vi "PicoScope6000ExampleStreaming.vi"() -> ()   [LabVIEW 2010]
doc: "This example demonstrates how to use the PicoScope Labview library to stream data from a PicoScope 5000 Series Device"
uses:
  PicoScope6000Lib/PicoScope6000AnalogChannelSettings.ctl
panel:
  in  "Write to file":bool
  in  "Trigger Settings":T1={"Trigger Enabled"=FALSE, "Trigger Source"=enum."Channel A", "Trigger Threshold (Volts)"=0.0, "Trigger Direction"=2, "Trigger Delay (samples)"=0, "Auto Trigger Time (ms)"=1000} {"Trigger Direction" items=["Rising"=2, "Falling"=3]}
  in  "error in (no error)":errorcluster
  out "Device Info":T2
  in  "Channel A Settings":T3={"Enabled"=TRUE, "Coupling"=1, "Range"=6, "Analogue Offset"=0.0, "Bandwidth"=0} {"Bandwidth" items=["Full", "20 MHz"]; "Range" items=["10 mV", "20 mV", "50 mV", "100 mV", "200 mV", "500 mV", "1 V", "2 V", "5 V", "10 V", "20 V", "50 V ", "100 V"]; "Coupling" items=["AC", "DC 1 MOhm", "DC 50 Ohm"]}
  out "Analog Channels":T4(graph)
  out "Raw Sample Interval (sec)":dbl=1.0000000130088963e-06 format="%#.5p"
  out "Max ADC value":i16=32512
  out "Chunk time":u32
  out "Elapsed time":dbl
  in  "Data file":path=path "PicoScope6000ExampleStreaming ChA Data"
  out "size(s)":i32
  out "Queue depth":i32(graph)
  out "queue depth":i32
  in  "Buffer and Transfer Settings":T5={"startIndex"=0, "Samples"=1000000, "Down Sample Ratio"=1, "Down-Sample Mode"=0} {"Down-Sample Mode" items=["None"=0, "Aggregate"=1, "Decimate"=2, "Average"=4]; "Down Sample Ratio" step=1; "Samples" format="%_6p"}
  out "TriggeredAt (In Buffer)":u32 format="%#.6p"
  out "TriggeredAt (Total samples)":u32 format="%#.6p"
  in  "Acquisition Settings":T6={"Auto Stop"=TRUE, "Desired Sample Interval"=1, "Pre-trigger Samples"=0, "Post-trigger Samples"=1000000, "Down-Sample Ratio"=1, "Down-Sample Mode"=0, "Time Units"=3} {"Time Units" items=["Nanoseconds (ns)"=2, "Microseconds (us)"=3, "Milliseconds (ms)"=4, "Seconds (s)"=5]; "Down-Sample Mode" items=["None"=0, "Aggregate"=1, "Decimate"=2, "Average"=4]; "Post-trigger Samples" format="%#.6p"; "Pre-trigger Samples" format="%#_6p"}
  out "Triggered":bool
  out "DownSample Interval (sec)":dbl=1.0000000130088963e-06 format="%#.5p"
  out "Total Samples":u32 format="%#.6p"
  out "Auto Stopped":bool
  in  "Serial Number":string
  in  "Open Using\nSerial Number":bool
  out "Number of Samples per Capture":u32 format="%#.6p"
  in  "Apply  Settings":bool
  in  "stop":bool
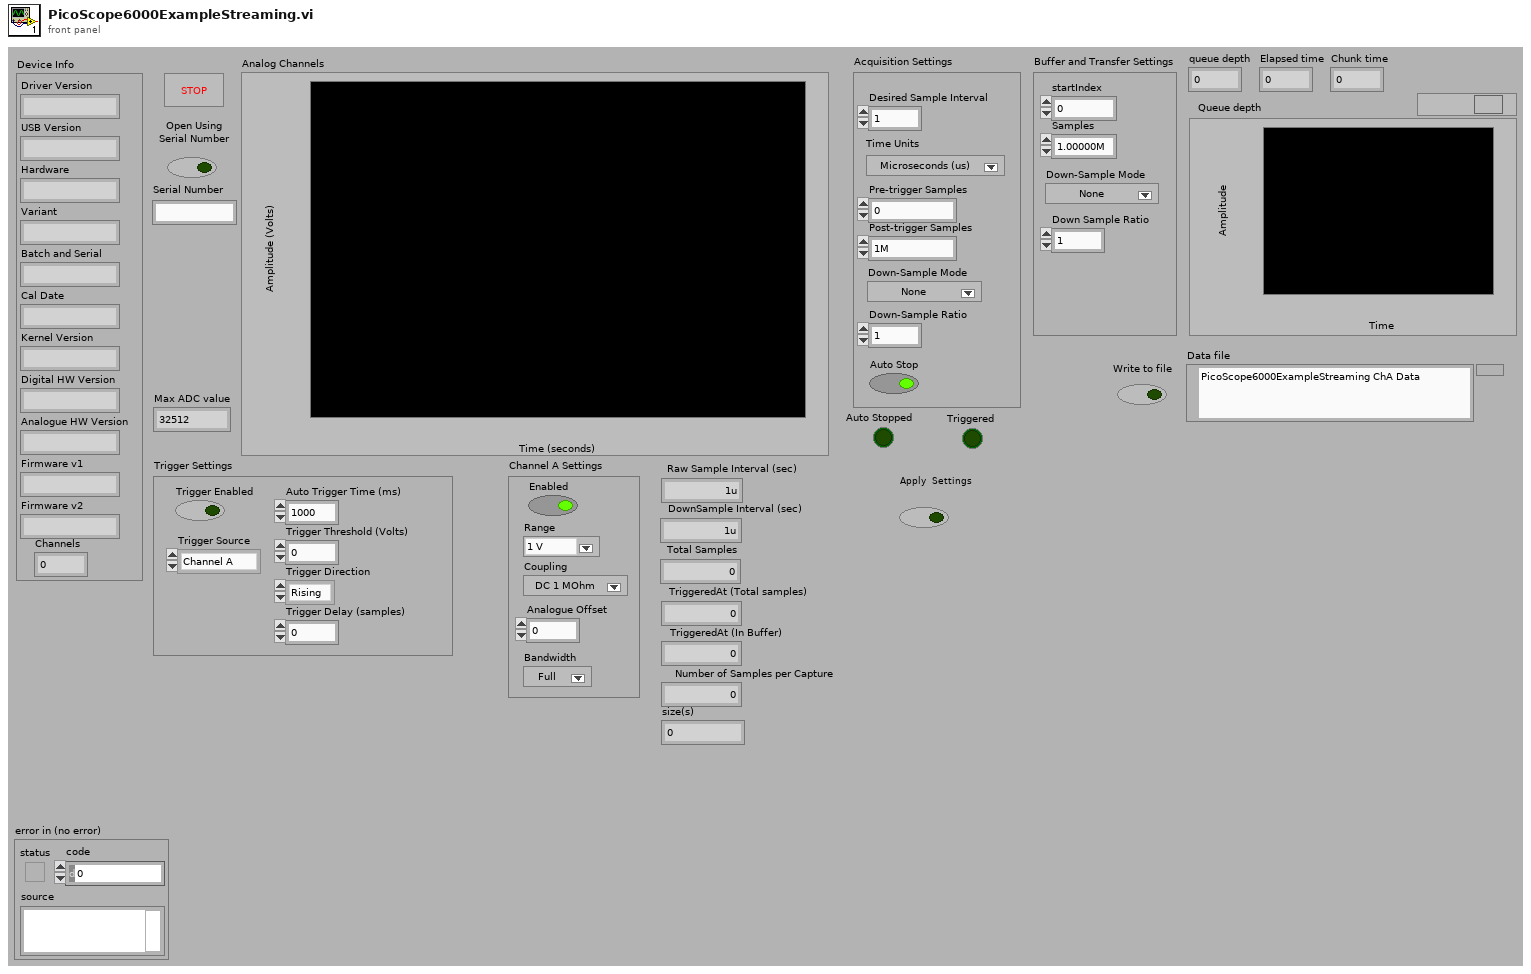
[diagram p1: front panel]
types:
  T1 = cluster{"Trigger Enabled":bool, "Trigger Source":enum32{"Channel A", "Channel B", "Channel C", "Channel D", "External", "Aux."}, "Trigger Threshold (Volts)":dbl, "Trigger Direction":u16, "Trigger Delay (samples)":u32, "Auto Trigger Time (ms)":i16}
  T2 = cluster{"Driver Version":string, "USB Version":string, "Hardware":string, "Variant":string, "Batch and Serial":string, "Cal Date":string, "Kernel Version":string, "Digital HW Version":string, "Analogue HW Version":string, "Firmware v1":string, "Firmware v2":string, "Channels":i16}
  T3 = typedef "PicoScope6000AnalogChannelSettings.ctl" = cluster{"Enabled":bool, "Coupling":u32, "Range":u32, "Analogue Offset":sgl, "Bandwidth":u32}
  T4 = cluster{i32, "DownSample Interval (sec)":dbl, "Data":dbl[]}
  T5 = cluster{"startIndex":u64, "Samples":u64, "Down Sample Ratio":u64, "Down-Sample Mode":u32}
  T6 = cluster{"Auto Stop":bool, "Desired Sample Interval":u32, "Pre-trigger Samples":u32, "Post-trigger Samples":u32, "Down-Sample Ratio":u32, "Down-Sample Mode":i32, "Time Units":u32}
  T7 = enum16{"open", "open or create", "create or replace", "create", "open (read-only)"}
  T8 = cluster{"Enabled":bool, "Coupling":i32, "Range":u16, "Analogue Offset":sgl, "Bandwidth":i32}
  T9 = cluster{"Channel A Buffer":i16[], "Channel B Buffer":i16[], "Channel C Buffer":i16[], "Channel D Buffer":i16[], "Channel E Buffer":i16[], "Channel F Buffer":i16[], "Channel G Buffer":i16[], "Channel H Buffer":i16[], "Port 0":i16[], "Port 1":i16[]}
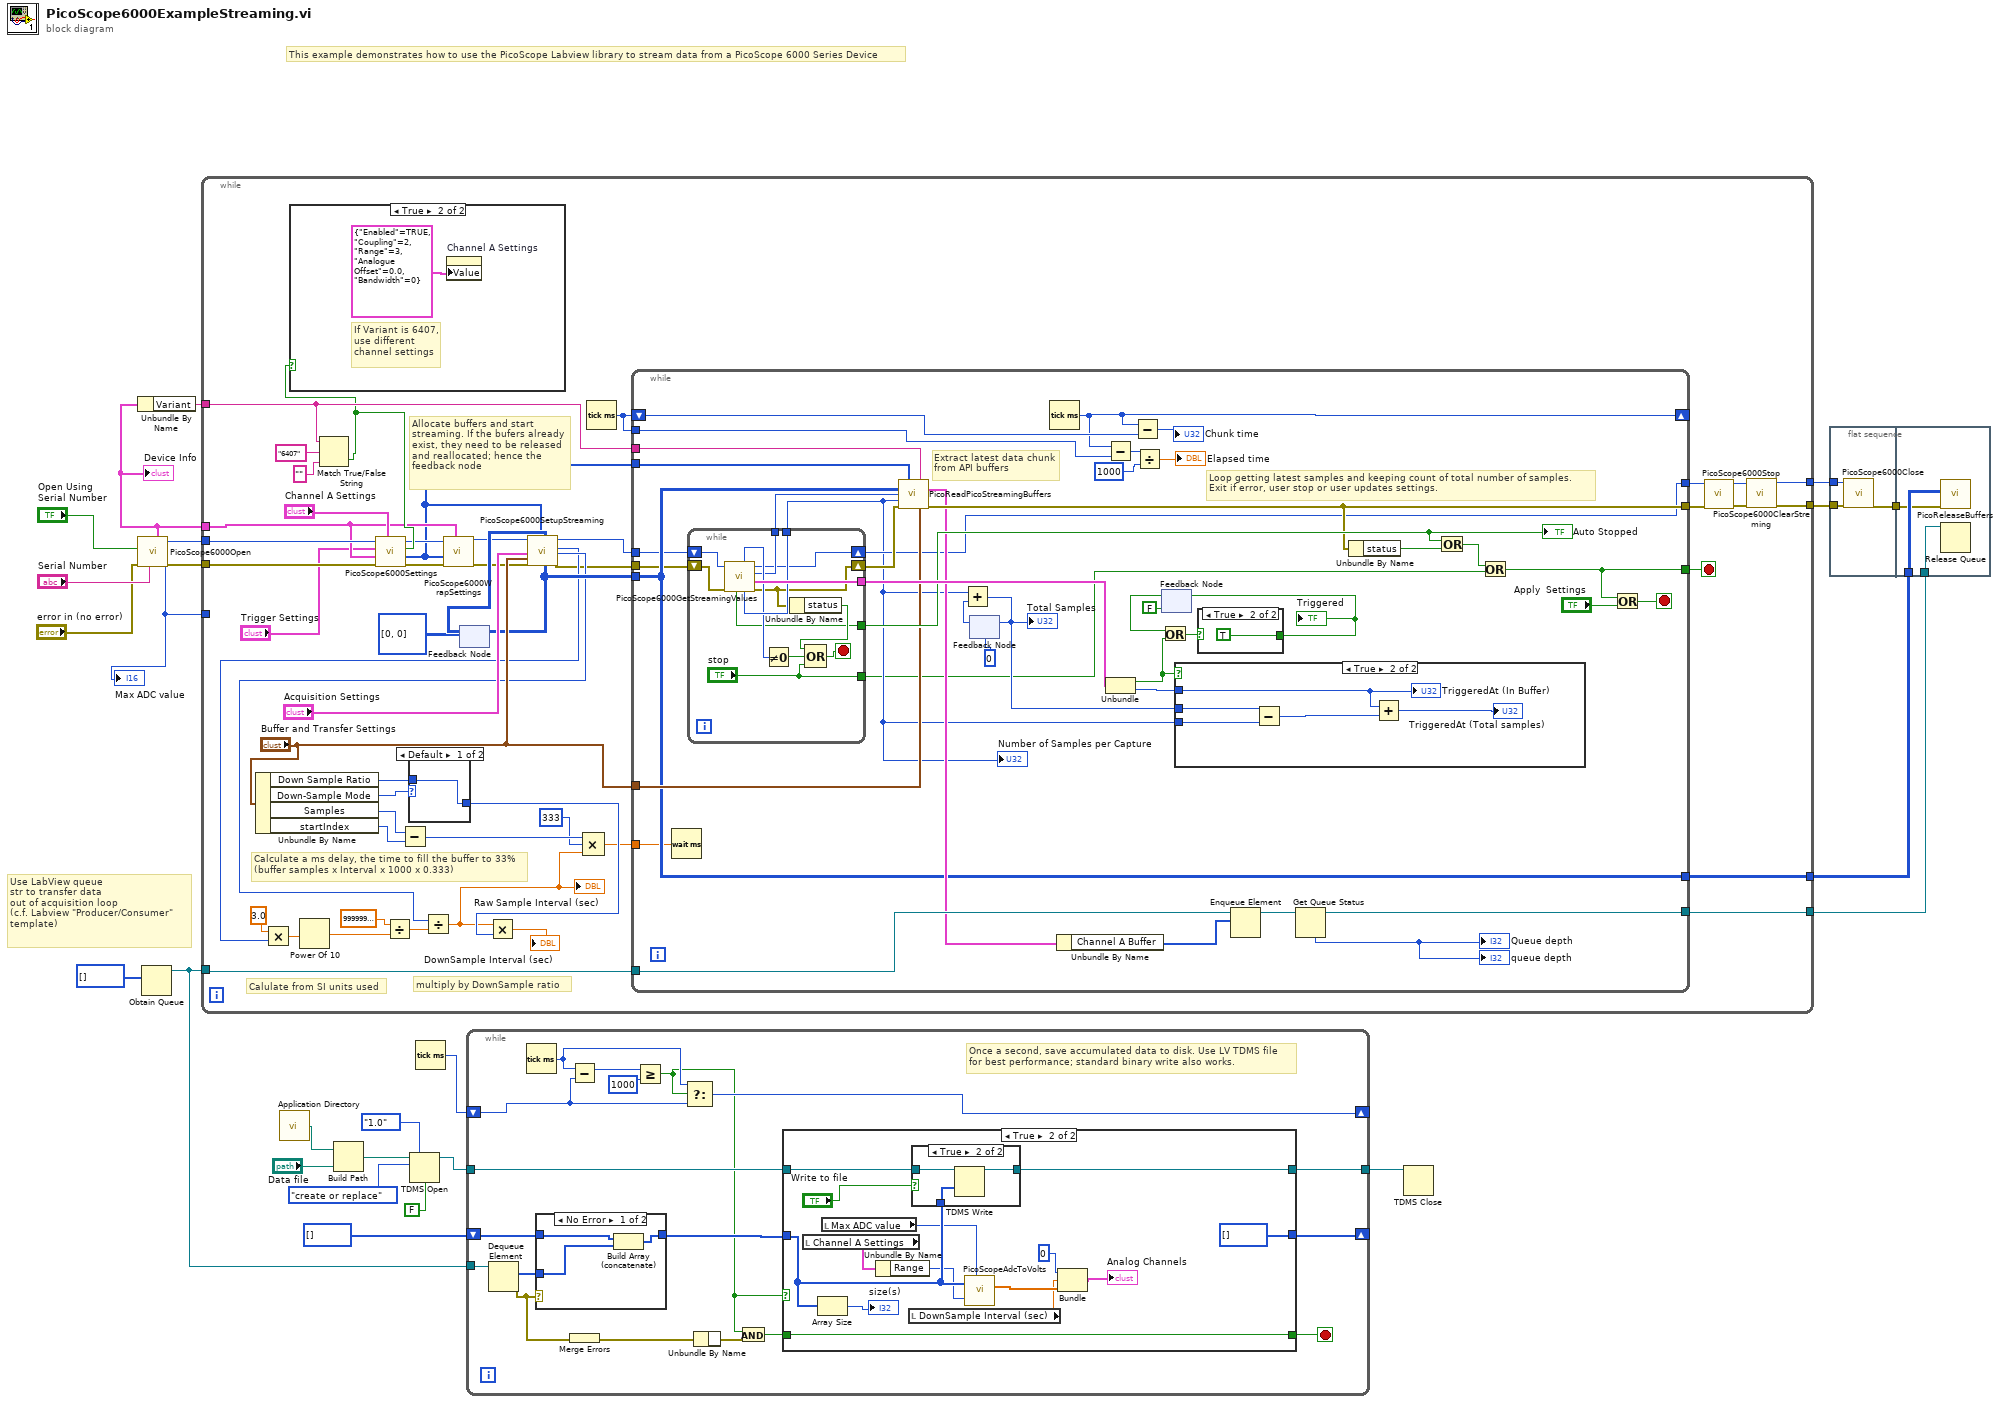
[diagram p0: block diagram]
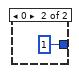
[diagram p6: hidden frame]
diagram:
  # "Use LabView queue\nstr to transfer data\nout of acquisition loop\n(c.f. Labview \"Producer/Consumer\"\ntemplate)"
  # "This example demonstrates how to use the PicoScope Labview library to stream data from a PicoScope 6000 Series Device"
  n1 = call "PicoScope6000Open.vi"("error in (no error)"="error in (no error)", "Serial Number"="Serial Number", "Use Serial Number"="Open Using\nSerial Number") -> ("error out"=w25:errorcluster, "Max Adc value"=w21:i16, "handle"=w24:i16, "Device Info"=w4:T2)  [unwired: 4 in, 1 out]
  "Max ADC value" <- w21
  "Device Info" <- w4
  n2 = Unbundle By Name(w4) -> ("Variant"=w5:string)
  n3 = Obtain Queue(element data type=i16[] [] ("History Data")) -> (queue out=w20:refnum<queue>)  [unwired: 4 in, 2 out]
  n4 = while {
    tunnel: [w27] -> w19
    tunnel: w25 -> [w44]
    tunnel: w24 -> [w43]
    tunnel: w21 -> [_]
    tunnel: [w69] -> w17
    tunnel: w20 -> [w68]
    tunnel: [w67] -> w18
    tunnel: w5 -> [w60]
    tunnel: w4 -> [w41]
    tunnel: [w26] -> w2
    stop <- w74 stop-if-true
    # "Calculate a ms delay, the time to fill the buffer to 33%\n(buffer samples x Interval x 1000 x 0.333)"
    # "multiply by DownSample ratio"
    # "Calulate from SI units used"
    # "Allocate buffers and start\nstreaming. If the bufers already\nexist, they need to be released\nand reallocated; hence the\nfeedback node"
    n5 = Unbundle By Name("Buffer and Transfer Settings") -> ("Down Sample Ratio"=w72:u64, "Down-Sample Mode"=w73:u32, "Samples"=w58:u64, "startIndex"=w57:u64)
    n6 = Match True/False String(2:"" ("false string"), 3:"6407" ("true string"), 4:w60) -> (0:w42:bool)  [unwired: 1 out]
    n7 = case shown="True" w42 {
      frame False {
      }
      frame True {
        # "If Variant is 6407,\nuse different \nchannel settings"
        n8 = property on="Channel A Settings" class="Clust (strict)"("Value"=T8 {"Enabled"=TRUE, "Coupling"=2, "Range"=3, "Analogue Offset"=0.0, "Bandwidth"=0} ("Channel A Settings")) -> ()  [unwired: 2 in, 2 out]
      }
    }
    n9 = call "PicoScope6000Settings.vi"("PS6407?"=w42, "Channel A Settings"="Channel A Settings", "error in"=w44, "Device Info"=w41, "Trigger Settings"="Trigger Settings", "handle in"=w43) -> ("error out"=w39:errorcluster, "Enabled array"=w33:i16[], "handle out"=w38:i16)  [unwired: 3 in]
    n10 = Subtract(x=w58, y=w57) -> (x-y=w48:u64)
    n11 = case shown="Default" w73 {
      tunnel: [w76 u32 1 ("Down-Sample Ratio")] -> w50
      tunnel: w72 -> [w76 _]
      frame Default {
      }
      frame 0 {
      }
    }
    n12 = call "PicoScope6000WrapSettings.vi"("Device Info"=w41, "error in (no error)"=w39, "enabledChannels"=w33, "Handle In"=w38) -> ("error out"=w35:errorcluster, "Handle Out"=w34:i16)  [unwired: 6 in]
    n13 = feedback #1(u64[][] [[0], [0]] ("Pointer array")) -> (w66:u64[][])
    n14 = call "PicoScope6000SetupStreaming.vi"("handle in"=w34, "Acquisition Settings"="Acquisition Settings", "Buffer and Transfer Settings"="Buffer and Transfer Settings", "error in"=w35, "enabled array"=w33, "Pointers In"=w66) -> ("Pointer array"=w65:u64[][], "handle out"=w30:i16, "sampleIntervalTimeUnits"=w32:u32, "Sample Interval"=w49:u32, "error out"=w31:errorcluster)  [unwired: 9 in]
    n15 = Multiply(x=3.0, y=w32) -> (x*y=w55:dbl)
    n16 = Power Of 10(x=w55) -> (10^x=w54:dbl)
    n17 = Divide(x=sgl 1000000000000000.0 ("y"), y=w54) -> (x/y=w53:dbl)
    n18 = Divide(x=w49, y=w53) -> (x/y=w46:dbl)
    "Raw Sample Interval (sec)" <- w46
    n19 = feedback-in #1(w65) -> ()
    n20 = Multiply(x=w46, y=w50) -> (x*y=→"DownSample Interval (sec)":dbl)
    n21 = Compound Arithmetic op=MULTIPLY(w48, u64 333 ("value"), w46) -> (w45:dbl)
    n22 = Tick Count (ms)() -> (millisecond timer value=w59:u32)
    n23 = while {
      tunnel: [w87] -> w36
      tunnel: [w118] -> w74
      tunnel: [w101] -> w37
      tunnel: "Buffer and Transfer Settings" -> [w103]
      tunnel: w33 -> [w100]
      tunnel: [w98] -> w69
      tunnel: w68 -> [w96]
      tunnel: w65 -> [w94]
      tunnel: [w94] -> w67
      shift-right: [w89] -> _
      shift-left: w59 -> [w90]
      tunnel: w60 -> [w84]
      tunnel: w59 -> [w81]
      tunnel: w45 -> [w80]
      tunnel: w31 -> [w79]
      tunnel: w30 -> [w78]
      stop <- w117 stop-if-true
      # "Loop getting latest samples and keeping count of total number of samples. \nExit if error, user stop or user updates settings."
      # "Extract latest data chunk\nfrom API buffers"
      n24 = Wait (ms)(milliseconds to wait=w80) -> ()  [unwired: 1 out]
      n25 = while {
        tunnel: [w132] -> w116
        tunnel: [w125] -> w113
        tunnel: [w124] -> w86
        tunnel: [w131] -> w85
        shift-right: [w123] -> w87
        shift-left: w78 -> [w122]
        shift-right: [w120] -> w102
        shift-left: w79 -> [w121]
        tunnel: ["stop"] -> w83
        stop <- w127 stop-if-true
        n26 = call "PicoScope6000GetStreamingValues.vi"("error in"=w121, "handle in"=w122) -> ("error out"=w120:errorcluster, "Trigger"=w132:cluster{bool, "triggeredAt":u32}, "Start Index"=w124:u32, "handle out"=w123:i16, "Number of Samples"=w131:u32, "ready"=w130:i16, "Auto Stopped"=w125:bool)  [unwired: 3 in]
        n27 = Not Equal To 0?(x=w130) -> (x != 0?=w128:bool)
        n28 = Unbundle By Name(w120) -> ("status"=w129:bool)
        n29 = Compound Arithmetic op=OR(w129, w128, "stop") -> (w127:bool)
      }
      "Number of Samples per Capture" <- w85
      "Auto Stopped" <- w113
      n30 = call "PicoReadPicoStreamingBuffers.vi"("enabled array"=w100, "Buffer and Transfer Settings"=w103, "Variant"=w84, "Pointer array"=w94, "Offset Index"=w86, "Number of Samples"=w85, "error in (no error)"=w102) -> ("Buffers (Max or non-aggregated)"=w95:T9, "error out"=w101:errorcluster)  [unwired: 6 in, 1 out]
      n31 = feedback #2(u32 0) -> (w109:u32)
      n32 = Add(x=w85, y=w109) -> (x+y=w107:u32)
      "Total Samples" <- w107
      n33 = feedback-in #2(w107) -> ()
      n34 = Tick Count (ms)() -> (millisecond timer value=w89:u32)
      n35 = Unbundle By Name(w95) -> ("Channel A Buffer"=w82:i16[])
      n36 = Subtract(x=w89, y=w81) -> (x-y=w93:u32)
      n37 = Unbundle(w116) -> (w105:bool, "triggeredAt"=w104:u32)
      n38 = Subtract(x=w89, y=w90) -> (x-y=→"Chunk time":u32)
      n39 = Divide(x=w93, y=u32 1000) -> (x/y=→"Elapsed time":dbl)
      n40 = feedback #3(FALSE) -> (w111:bool)
      n41 = Or(x=w111, y=w105) -> (x .or. y?=w108:bool)
      n42 = case shown="True" w105 {
        tunnel: w85 -> [_ w133]
        tunnel: w107 -> [_ w137]
        tunnel: w104 -> [_ w135]
        frame False {
        }
        frame True {
          n43 = Subtract(x=w137, y=w133) -> (x-y=w136:u32)
          n44 = Add(x=w135, y=w136) -> (x+y=→"TriggeredAt (Total samples)":u32)
          "TriggeredAt (In Buffer)" <- w135
        }
      }
      n45 = case shown="True" w108 {
        selector: w108 -> [w138 _]
        tunnel: [w138 TRUE] -> w106
        frame False {
        }
        frame True {
        }
      }
      "Triggered" <- w106
      n46 = feedback-in #3(w106) -> ()
      n47 = Enqueue Element(queue=w96, element=w82) -> (queue out=w97:refnum<queue>)  [unwired: 2 in, 2 out]
      n48 = Get Queue Status(queue=w97) -> (queue out=w98:refnum<queue>, # elements in queue=→"queue depth" →"Queue depth":i32)  [unwired: 2 in, 6 out]
      n49 = Unbundle By Name(w101) -> ("status"=w115:bool)
      n50 = Or(x=w113, y=w115) -> (x .or. y?=w114:bool)
      n51 = Or(x=w114, y=w83) -> (x .or. y?=w118:bool)
      n52 = Or(x=w118, y="Apply  Settings") -> (x .or. y?=w117:bool)
    }
    n53 = call "PicoScope6000Stop.vi"("error in (no error)"=w37, "handle"=w36) -> ("error out"=w29:errorcluster, "handle out"=w28:i16)  [unwired: 8 in]
    n54 = call "PicoScope6000ClearStreming.vi"("error in (no error)"=w29, "handle"=w28) -> ("error out"=w26:errorcluster, "handle out"=w27:i16)  [unwired: 8 in]
  }
  n55 = call <vilib>:"Application Directory.vi"() -> ("Application Directory"=w6:path)
  n56 = Build Path(base path=w6, name or relative path="Data file") -> (appended path=w7:path)
  n57 = TDMS Open(6:FALSE ("disable buffering? (T)"), 7:enum16{"1.0", "2.0"}."1.0" ("file format version (2.0)"), 10:T7."create or replace" ("operation (0:open)"), 11:w7) -> (3:w14:refnum<k34>)  [unwired: 2 in, 1 out]
  n58 = Tick Count (ms)() -> (millisecond timer value=w16:u32)
  n59 = while {
    tunnel: w20 -> [w156]
    shift-right: [w149] -> _
    shift-left: i16[] [] ("History Data") -> [w155]
    shift-right: [w150] -> _
    shift-left: w16 -> [w151]
    tunnel: w14 -> [w148]
    tunnel: [w147] -> w13
    stop <- w142 stop-if-true
    # "Once a second, save accumulated data to disk. Use LV TDMS file\nfor best performance; standard binary write also works."
    n60 = Dequeue Element(queue=w156) -> (element=w157:i16[], error out=w146:errorcluster)  [unwired: 2 in, 2 out]
    n61 = Tick Count (ms)() -> (millisecond timer value=w152:u32)
    n62 = case shown="No Error" w146 {
      tunnel: w155 -> [w180 w181]
      tunnel: [w179 w181] -> w145
      tunnel: w157 -> [w178 _]
      frame No Error {
        n63 = Build Array (concatenate)(w180, w178) -> (w179:i16[])
      }
      frame Error {
      }
    }
    n64 = Subtract(x=w152, y=w151) -> (x-y=w154:u32)
    n65 = Merge Errors(w146) -> (w143:errorcluster)
    n66 = Greater Or Equal?(x=w154, y=u32 1000) -> (x >= y?=w141:bool)
    n67 = Select(t=w152, s=w141, f=w151) -> (s? t:f=w150:u32)
    n68 = And(x=w141) -> (y=w140:errorcluster, x .and. y?=w144:bool)
    n69 = Unbundle By Name(w143, w140) -> ()
    n70 = case shown="True" w141 {
      tunnel: w145 -> [w159 w169]
      tunnel: [w159 i16[] [] ("History Data")] -> w149
      tunnel: w148 -> [w158 w171]
      tunnel: [w158 w170] -> w147
      tunnel: [_ w161] -> w142
      tunnel: w144 -> [_ w161]
      frame False {
      }
      frame True {
        n71 = local read "Channel A Settings"() -> (w162:T3)
        n72 = Array Size(array=w169) -> (size(s)=→"size(s)":i32)
        n73 = local read "Max ADC value"() -> (w165:i16)
        n74 = Unbundle By Name(w162) -> ("Range"=w168:u32)
        n75 = local read "DownSample Interval (sec)"() -> (w164:dbl)
        n76 = case shown="True" "Write to file" {
          tunnel: w171 -> [w174 w177]
          tunnel: [w174 w176] -> w170
          tunnel: w169 -> [_ w175]
          frame False {
          }
          frame True {
            n77 = TDMS Write(0:w177, 9:w175) -> (4:w176:refnum<k34>)  [unwired: 4 in, 3 out]
          }
        }
        n78 = call "PicoScopeAdcToVolts.vi"("Max_adc"=w165, "Range Index"=w168, "Data"=w169) -> ("Data"=w166:dbl[])
        n79 = Bundle(0, "DownSample Interval (sec)"=w164, "Data"=w166) -> (→"Analog Channels":T4)  [unwired: 1 in]
      }
    }
  }
  n80 = TDMS Close(11:w13) -> ()  [unwired: 1 in, 2 out]
  n81 = flat-sequence {
    tunnel: w19 -> [w184]
    tunnel: w2 -> [w183]
    tunnel: [w182] -> w1
    tunnel: w18 -> [w187]
    tunnel: w17 -> [w186]
    tunnel: w1 -> [w185]
    frame #0 {
      n82 = call "PicoScope6000Close.vi"("error in (no error)"=w183, "handle"=w184) -> ("error out"=w182:errorcluster)  [unwired: 8 in, 1 out]
    }
    frame #1 {
      n83 = call "PicoReleaseBuffers.vi"("error in (no error)"=w185, "Pointer array"=w187) -> ()  [unwired: 8 in, 2 out]
      n84 = Release Queue(queue=w186) -> ()  [unwired: 2 in, 3 out]
    }
  }
